vi "VNAconsole.vi"() -> ()   [LabVIEW 2017]
uses:
  ScanTarget.ctl
  ScanPara.ctl
  Action.ctl
  InstrPara.ctl
  <vilib>/Utility/xml.llb/Write to XML File(string).vi
  <vilib>/Utility/xml.llb/Read From XML File(string).vi
  <vilib>/Utility/file.llb/Write Delimited Spreadsheet (DBL).vi
  <instrlib>/Agilent ENA Series/Agilent ENA Series.lvlib
  <instrlib>/Agilent PNA Series/Agilent PNA Series.lvlib
panel:
  out "CrntScan 2":dbl[](array[numeric]) caption="Current scan"
  in  "Panel":enum32{"Meas", "Graph"}(tab)
  out "TimeLeft":dbl
  in  "ThermalizationTime":dbl=600.0 caption="Settling\nTime (sec)"
  in  "FAA_SetT":dbl caption="FAA  Set T(K)\n ADR  0=off" min=0.0 max=10.0
  in  "LoadSettings":bool caption="Load settings?"
  in  "SettingsPath":path=path "O:/68707/BF2222/LABVIEWdata/VNA" caption="Settings path"
  in  "Comment":string
  in  "Config":enum32{"PNA", "ENA"}(tab)
  in  "PNA Config":T1={"Sweep Type"=0, "Sweep Gen Type"=0, "Sweep Points"=32001, "Bandwidth (Hz)"=1000.0, "Center Freq (Hz)"=25005000000.0, "Span Freq (Hz)"=49990000000.0, "Power Level (dBm)"=-87.0, "Average Count"=1, "Electrical Delay (s)"=0.0} {"Electrical Delay (s)" min=0.0 max=1000000000.0 format="%.6p"; "Average Count" min=1 max=65536 step=1; "Power Level (dBm)" min=-87.0 max=10.0 format="%.2p"; "Span Freq (Hz)" min=0.0 max=49990000000.0 format="%.6p"; "Center Freq (Hz)" min=10000000.0 max=50000000000.0 format="%.6p"; "Bandwidth (Hz)" min=1.0 max=40000.0 format="%.2p"; "Sweep Points" min=1 max=32001 step=1; "Sweep Gen Type" items=["Analog", "Stepped"]; "Sweep Type" items=["Linear Frequency", "Log Frequency", "Power Sweep", "CW Time"]}
  in  "ENAConfig":T2={"Sweep Type"=0, "Sweep Mode"=1, "Sweep Points"=3201, "Average count"=1, "IF Bandwidth (Hz)"=1000.0, "Power Level (dBm)"=-85.0, "Center Freq (Hz)"=10000150000.0, "Span Freq (Hz)"=19999700000.0, "Electrical Delay (s)"=0.0} caption="ENA Config" {"Electrical Delay (s)" min=0.0 max=10.0 format="%.2p"; "Span Freq (Hz)" min=0.0 max=19999700000.0 format="%.6p"; "Center Freq (Hz)" min=300000.0 max=20000000000.0 format="%.6p"; "Power Level (dBm)" min=-85.0 max=10.0 format="%^.2g"; "IF Bandwidth (Hz)" min=10.0 max=1500000.0 format="%.1p"; "Average count" min=1 max=999 step=1; "Sweep Points" min=1 max=3201 step=1; "Sweep Mode" items=["Stepped", "Swept", "Fast Stepped Mode", "Fast Swept Mode"]; "Sweep Type" items=["Linear Sweep", "Logarithmic Sweep", "Segment Sweep", "Power Sweep", "DC Bias"]}
  in  "Run":bool caption="Run?"
  in  "Scans":T5(array[cluster])=[{"Target"=enum."VNA", "Parameter"=enum."N.A.", "Start"=0.0, "Stop"=0.0, "#Steps"=1, "ScanArray"=[0.0]}] {"Stop" format="%.9f"; "Start" format="%.9f"; "#Steps" min=1 step=1}
  in  "SYS":T6={"ScanStep"=[], "ScanSizes"=[], "Data Path"=path "C:/data", "Scans"=[], "GPIB_ENA"="GPIB0::17::INSTR", "Savingfolder"=path "", "GPIB_PNA"="GPIB0::16::INSTR", "PhysCH"={"Fridge"="ADR", "VNA"="PNA #E8364C"}, "GPIB_PPMS"="GPIB0::15::INSTR"} {"Scans"."Stop" format="%.9f"; "Scans"."Start" format="%.9f"}
  out "VNA Data":dbl[][](array[numeric])
  out "VNA Freq":dbl[](array[numeric])
  out "Routing":variant=variant(enum16{"Startup", "Shutdown", "SaveSettings", "LoadSettings", "InitVNA", "CloseVNA", "InitScan", "IncrementScan", "StopScan", "Target=VNA", "Acquire", "Graph", "PNA", "ENA"} enum."Graph")
  in  "Acquiring":bool
  out "Shutdown":bool=TRUE
  in  "Meas":T7={"S11"=FALSE, "S12"=FALSE, "S21"=TRUE, "S22"=FALSE}
  out "T_status":string caption="Temperature Status"
  out "FinalT":dbl
  out "ENA Mag":cluster{dbl[], "Data":dbl[]}[](graph) caption="ENA Magnitude"
  out "ENA Phz":cluster{dbl[], "Data":dbl[]}[](graph) caption="ENA Phase"
  out "CrntScan":dbl[](array[numeric]) caption="Current scan"
  out "XY Graph":cluster{"all rows":dbl[], dbl[]}[](graph)
  out "rotated and translated circle":cluster{dbl[], dbl[]}(graph)
  out "Fits":T8 {"Q_i" format="%#.0f"; "Q_c" format="%#.0f"; "Q_r" format="%#1.0f"; "f_r" format="%#_9p"}
  # "Target"
  # "Parameter"
  # "Start"
  # "Stop"
  # "Yellow fields are controls.\nBlue fields are indicators.\nCheck all yellow fields before RUN.\nScans override Config."
  # "#Steps"
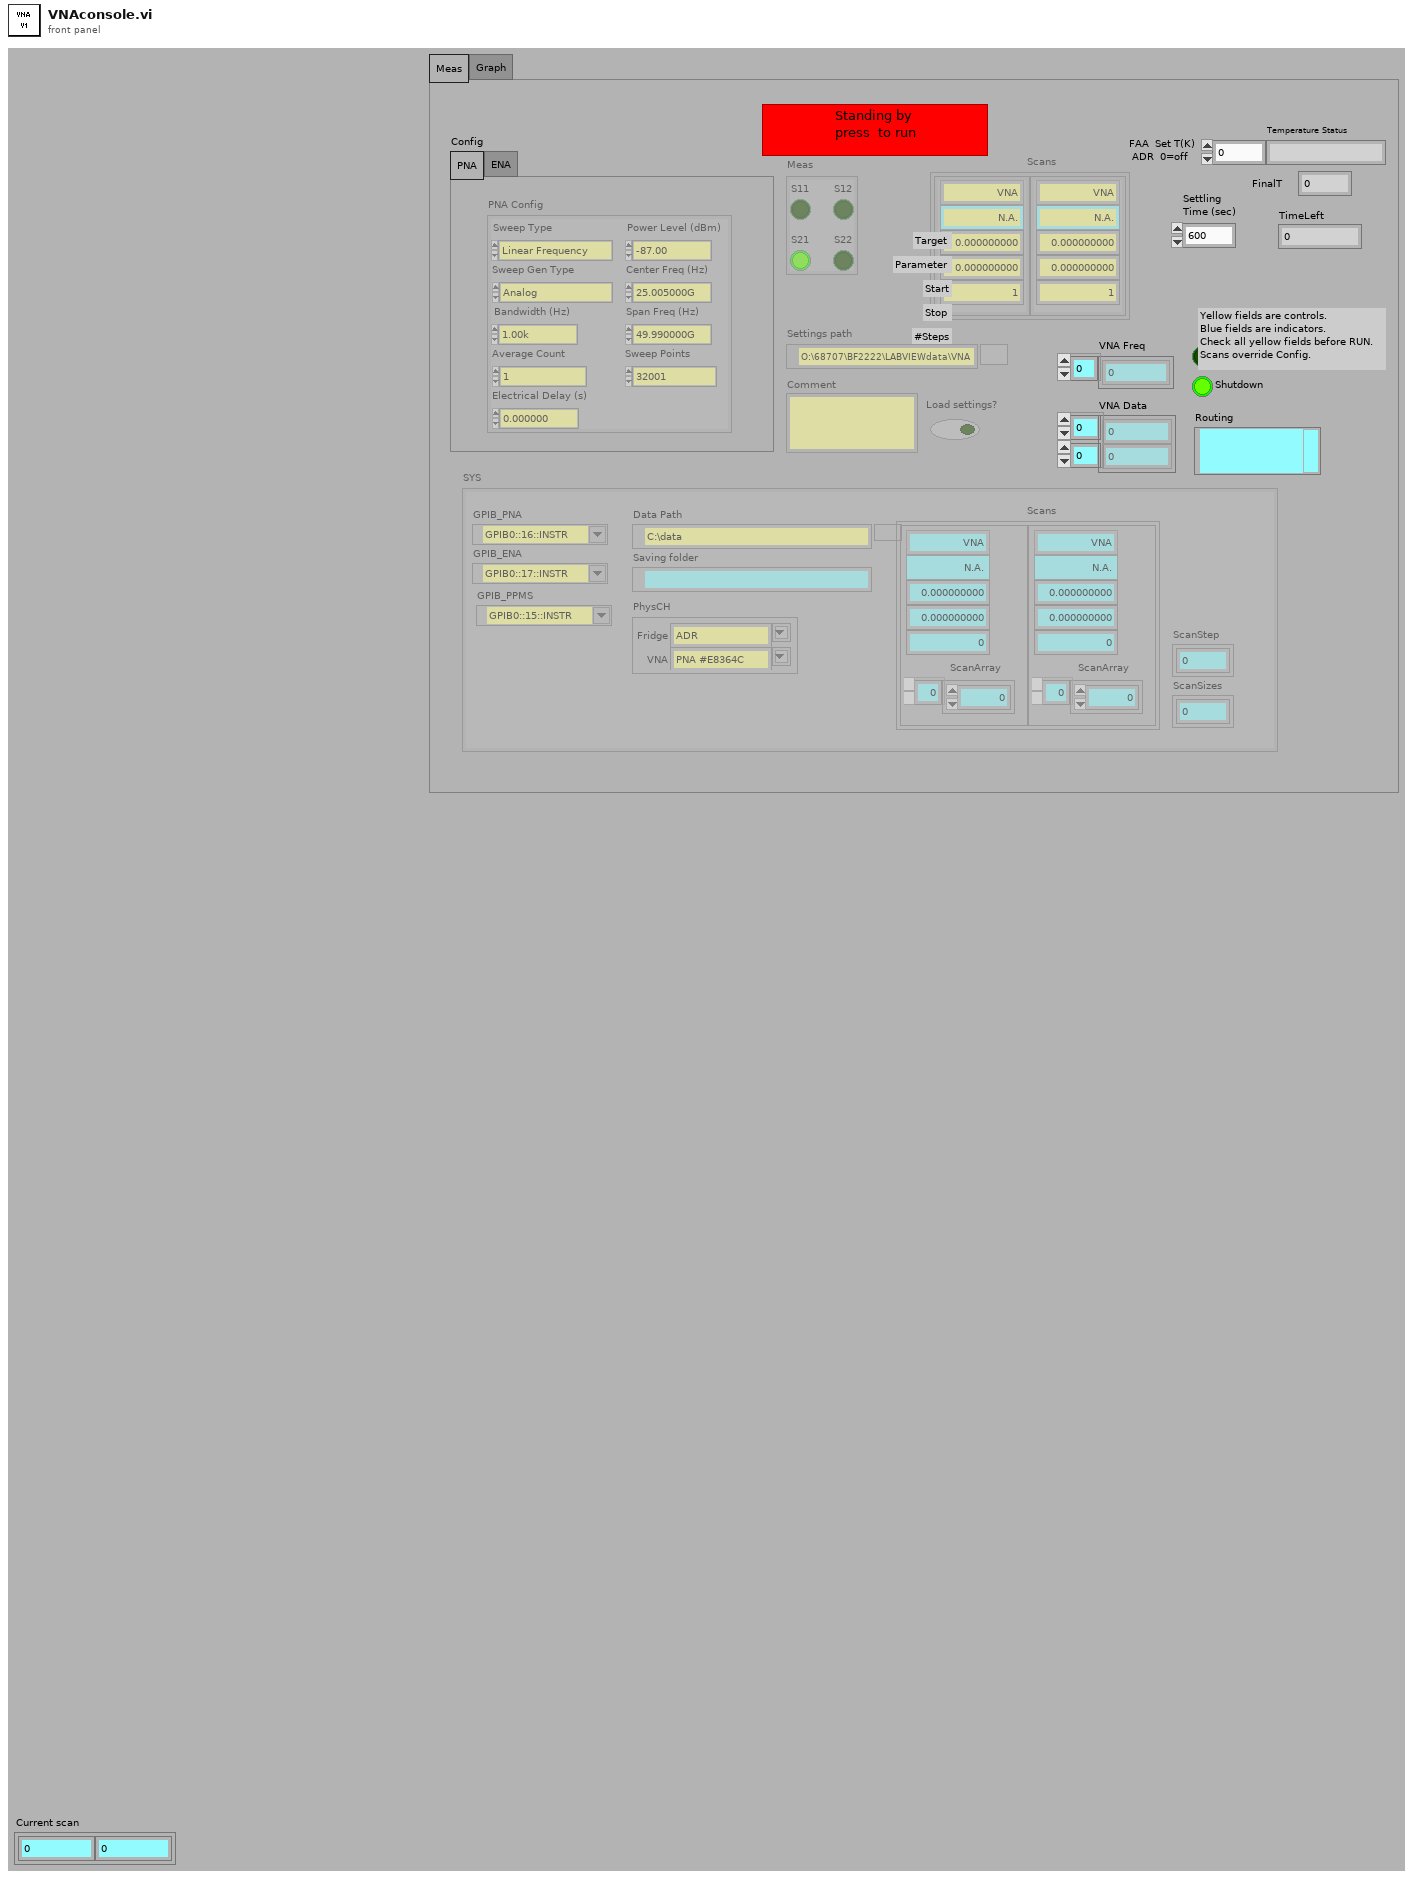
[diagram p1: front panel]
types:
  T1 = cluster{"Sweep Type":i32, "Sweep Gen Type":i32, "Sweep Points":i32, "Bandwidth (Hz)":dbl, "Center Freq (Hz)":dbl, "Span Freq (Hz)":dbl, "Power Level (dBm)":dbl, "Average Count":i32, "Electrical Delay (s)":dbl}
  T2 = cluster{"Sweep Type":u16, "Sweep Mode":u16, "Sweep Points":i32, "Average count":i32, "IF Bandwidth (Hz)":dbl, "Power Level (dBm)":dbl, "Center Freq (Hz)":dbl, "Span Freq (Hz)":dbl, "Electrical Delay (s)":dbl}
  T3 = typedef "ScanTarget.ctl" = enum16{"VNA", "Refrigerator"}
  T4 = typedef "ScanPara.ctl" = enum16{"Freq (GHz)", "Pwr (dBm)", "Temp (K)", "N.A."}
  T5 = cluster{"Target":T3, "Parameter":T4, "Start":dbl, "Stop":dbl, "#Steps":u32, "ScanArray":dbl[]}[]
  T6 = cluster{"ScanStep":i32[], "ScanSizes":i32[], "Data Path":path, "Scans":cluster{"Target":T3, "Parameter":T4, "Start":dbl, "Stop":dbl, "#Steps":u32, "ScanArray":dbl[]}[], "GPIB_ENA":refnum<visa-resource-name>, "Savingfolder":path, "GPIB_PNA":refnum<visa-resource-name>, "PhysCH":cluster{"Fridge":string, "VNA":string}, "GPIB_PPMS":refnum<visa-resource-name>}
  T7 = cluster{"S11":bool, "S12":bool, "S21":bool, "S22":bool}
  T8 = cluster{"f_r":dbl, "Q_r":dbl, "Q_c":dbl, "Q_i":dbl, "angle":dbl, "residue":dbl}
  T9 = typedef "Action.ctl" = enum16{"Startup", "Shutdown", "SaveSettings", "LoadSettings", "InitVNA", "CloseVNA", "InitScan", "IncrementScan", "StopScan", "Target=VNA", "Target=Refrigerator", "Acquire", "Graph", "PNA", "ENA", "ADR", "PPMS"}
  T10 = typedef "Semaphore RefNum" = refnum<k1>
  T11 = typedef "InstrPara.ctl" = cluster{"Parameter":string, "Channel":i32, "Instr#":i32, "Settings":variant}
  T12 = cluster{"PNA Config":cluster{"Sweep Type":i32, "Sweep Gen Type":i32, "Sweep Points":i32, "Bandwidth (Hz)":dbl, "Center Freq (Hz)":dbl, "Span Freq (Hz)":dbl, "Power Level (dBm)":dbl, "Average Count":i32, "Electrical Delay (s)":dbl}, "Meas":cluster{"S11":bool, "S12":bool, "S21":bool, "S22":bool}}
  T13 = cluster{"ENAConfig":cluster{"Sweep Type":u16, "Sweep Mode":u16, "Sweep Points":i32, "Average count":i32, "IF Bandwidth (Hz)":dbl, "Power Level (dBm)":dbl, "Center Freq (Hz)":dbl, "Span Freq (Hz)":dbl, "Electrical Delay (s)":dbl}, "Meas":cluster{"S11":bool, "S12":bool, "S21":bool, "S22":bool}}
  T14 = enum8{"Enabled", "Disabled", "Disabled and Grayed Out"}
  T15 = cluster{"Scans":cluster{"Scans":cluster{"Target":T3, "Parameter":T4, "Start":dbl, "Stop":dbl, "#Steps":u32, "ScanArray":dbl[]}[], "ScanSizes":i32[]}, "VNA":cluster{"PNA Config":cluster{"Sweep Type":i32, "Sweep Gen Type":i32, "Sweep Points":i32, "Bandwidth (Hz)":dbl, "Center Freq (Hz)":dbl, "Span Freq (Hz)":dbl, "Power Level (dBm)":dbl, "Average Count":i32, "Electrical Delay (s)":dbl}, "ENAConfig":cluster{"Sweep Type":u16, "Sweep Mode":u16, "Sweep Points":i32, "Average count":i32, "IF Bandwidth (Hz)":dbl, "Power Level (dBm)":dbl, "Center Freq (Hz)":dbl, "Span Freq (Hz)":dbl, "Electrical Delay (s)":dbl}, "Meas":cluster{"S11":bool, "S12":bool, "S21":bool, "S22":bool}}, "PhysCH":cluster{"Fridge":string, "VNA":string}, "Comment":string}
  T16 = cluster{"PNA Config":cluster{"Sweep Type":i32, "Sweep Gen Type":i32, "Sweep Points":i32, "Bandwidth (Hz)":dbl, "Center Freq (Hz)":dbl, "Span Freq (Hz)":dbl, "Power Level (dBm)":dbl, "Average Count":i32, "Electrical Delay (s)":dbl}, "ENAConfig":cluster{"Sweep Type":u16, "Sweep Mode":u16, "Sweep Points":i32, "Average count":i32, "IF Bandwidth (Hz)":dbl, "Power Level (dBm)":dbl, "Center Freq (Hz)":dbl, "Span Freq (Hz)":dbl, "Electrical Delay (s)":dbl}, "Meas":cluster{"S11":bool, "S12":bool, "S21":bool, "S22":bool}}
  T17 = cluster{"Scans":cluster{"Target":T3, "Parameter":T4, "Start":dbl, "Stop":dbl, "#Steps":u32, "ScanArray":dbl[]}[], "ScanSizes":i32[]}
  T18 = cluster{"PNA Config":variant, "Meas":cluster{"S11":bool, "S12":bool, "S21":bool, "S22":bool}}
  T19 = cluster{"Target":T3, "Parameter":T4, "Start":dbl, "Stop":dbl, "#Steps":u32, "ScanArray":dbl[]}
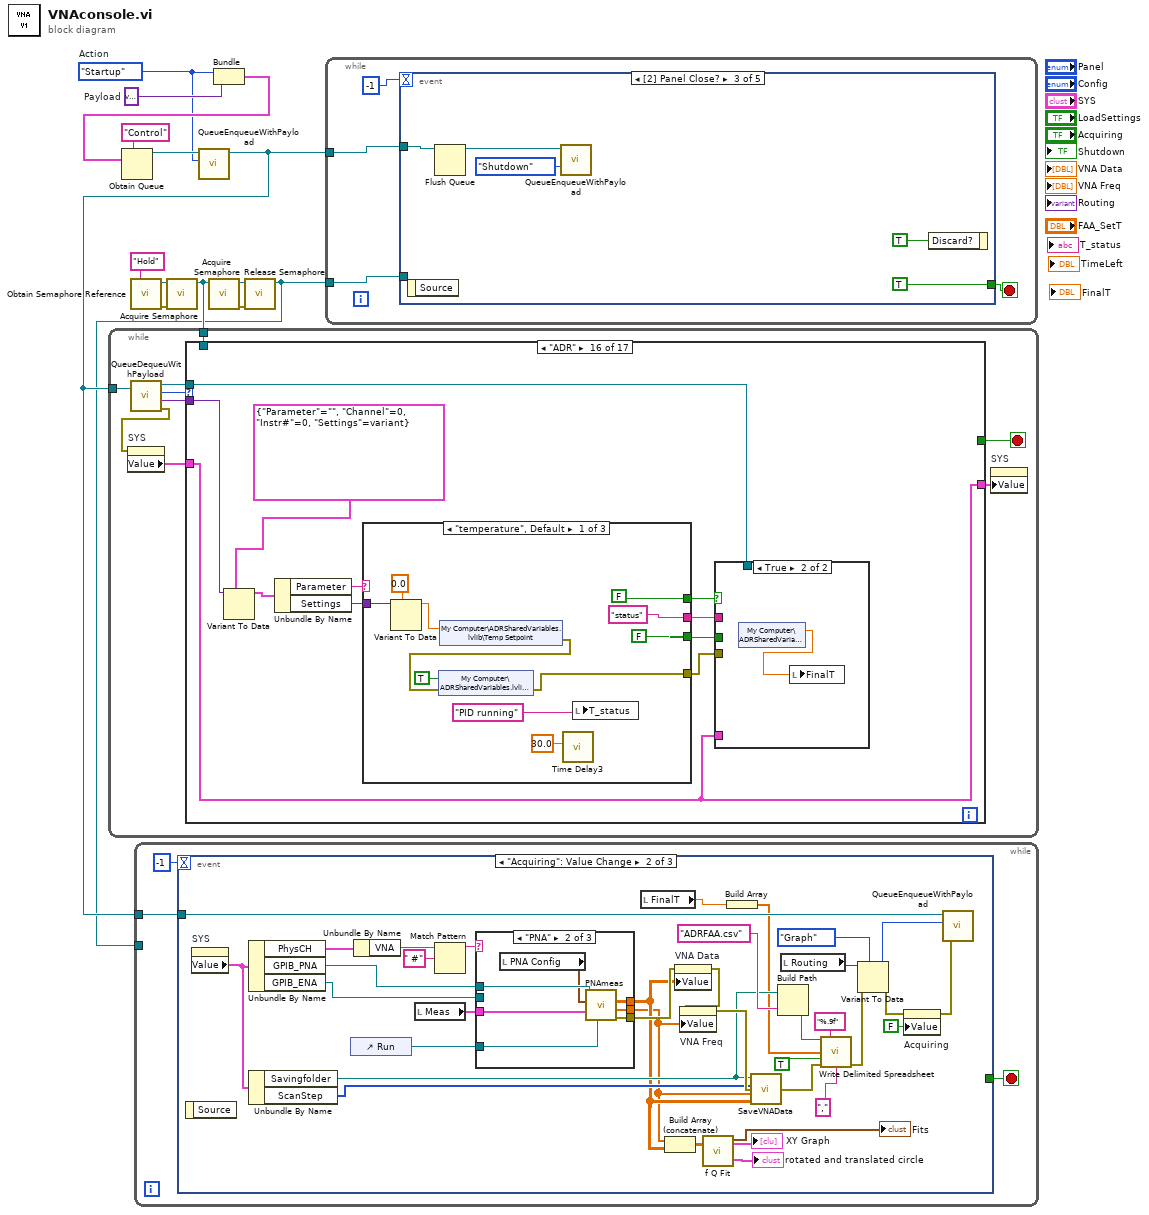
[diagram p0: block diagram]
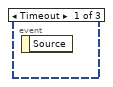
[diagram p2: hidden frame]
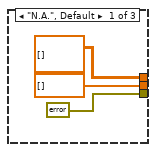
[diagram p3: hidden frame]
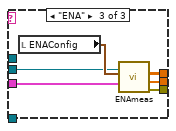
[diagram p4: hidden frame]
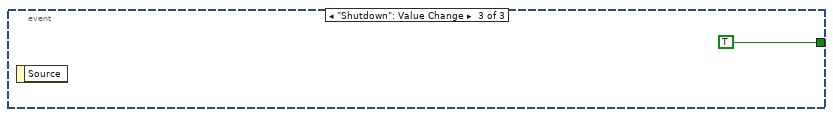
[diagram p5: hidden frame]
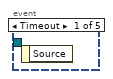
[diagram p6: hidden frame]
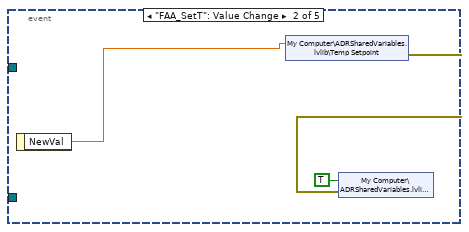
[diagram p7: hidden frame]
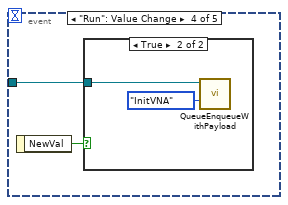
[diagram p8: hidden frame]
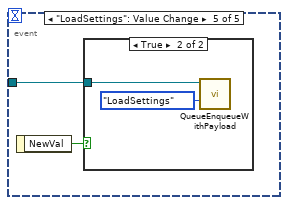
[diagram p10: hidden frame]
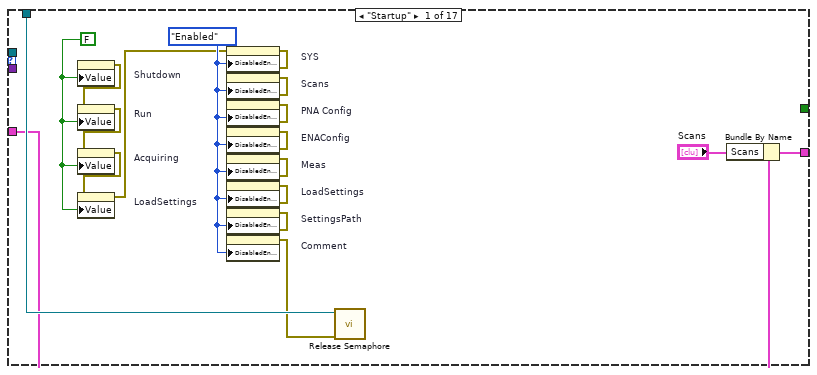
[diagram p12: hidden frame]
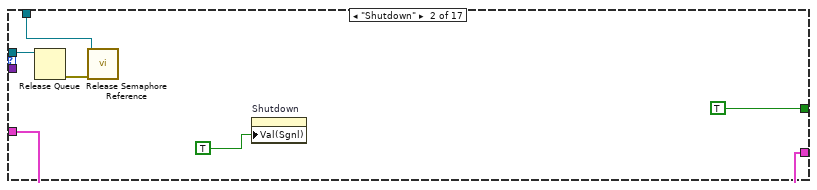
[diagram p13: hidden frame]
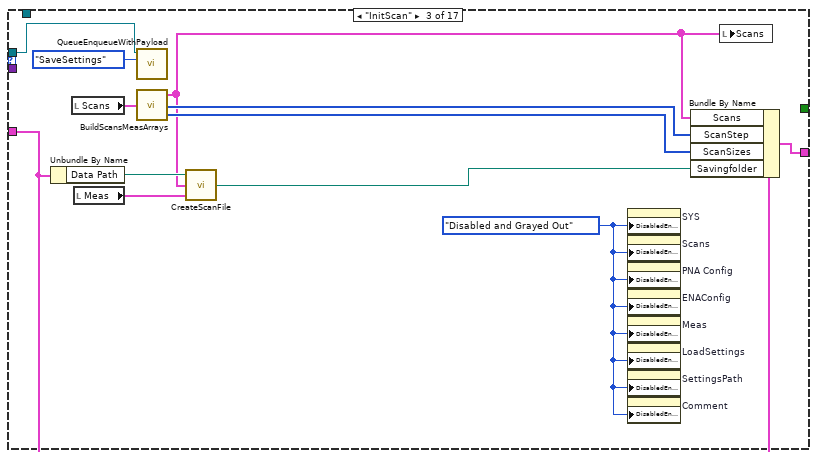
[diagram p14: hidden frame]
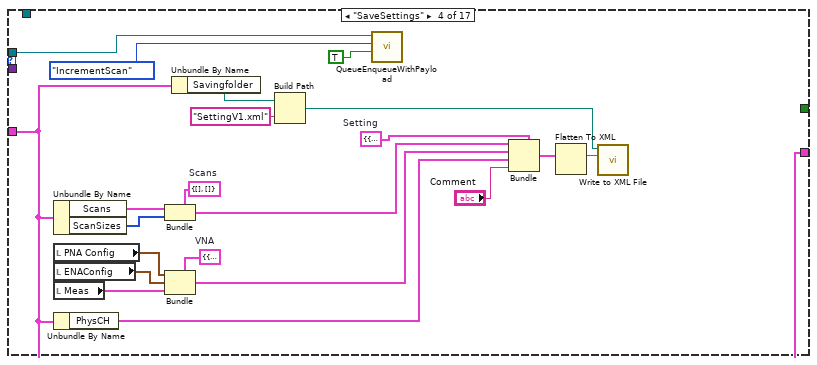
[diagram p15: hidden frame]
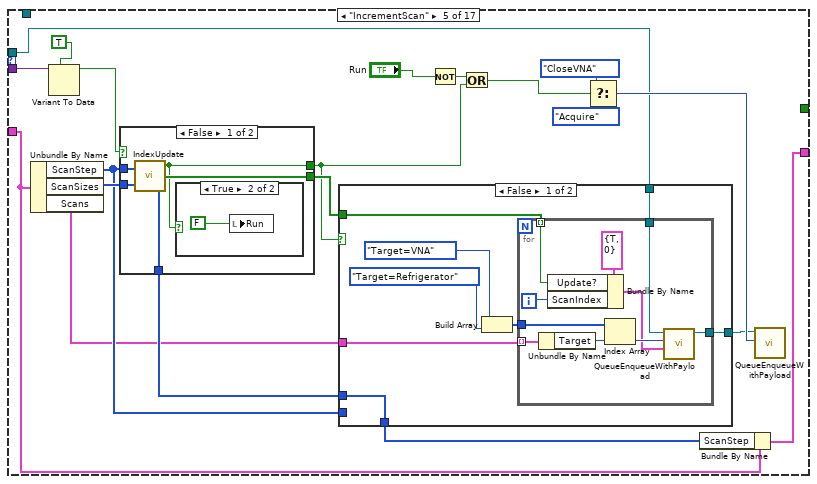
[diagram p16: hidden frame]
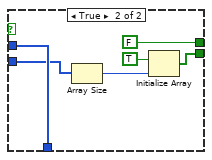
[diagram p19: hidden frame]
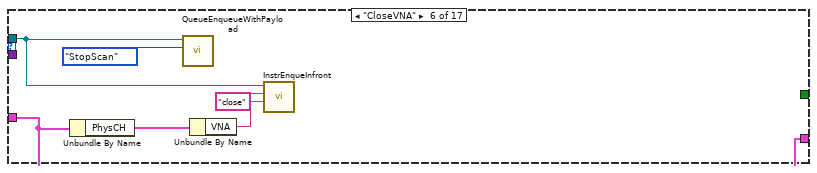
[diagram p20: hidden frame]
diagram:
  w6 = variant  # Payload
  w3 = Action."Startup"  # Action
  n1 = call <vilib>:"Obtain Semaphore Reference.vi"("name (unnamed)"="Hold") -> ("error out"=w11:errorcluster, "semaphore"=w10:T10)  [unwired: 4 in, 1 out]
  n2 = call <vilib>:"Acquire Semaphore.vi"("error in (no error)"=w11, "semaphore"=w10) -> ("semaphore out"=w9:T10)  [unwired: 3 in, 2 out]
  n3 = call <vilib>:"Acquire Semaphore.vi"("semaphore"=w9) -> ("error out"=w8:errorcluster, "semaphore out"=w7:T10)  [unwired: 4 in, 1 out]
  n4 = Bundle("Action"=w3, "Payload"=w6) -> (w5:cluster{"Action":T9, "Payload":variant})  [unwired: 1 in]
  n5 = Obtain Queue(name (unnamed)="Control", element data type=w5) -> (queue out=w4:refnum<queue>)  [unwired: 3 in, 2 out]
  n6 = call "QueueEnqueueWithPayload.vi"("Action"=w3, "Queue in"=w4) -> ("Queue out"=w2:refnum<queue>)  [unwired: 2 in, 1 out]
  n7 = while {
    tunnel: w2 -> [w16]
    tunnel: w9 -> [w21]
    stop <- w22 stop-if-true
    n8 = call "QueueDequeuWithPayload.vi"("Queue in"=w16) -> ("Queue out"=w17:refnum<queue>, "Action"=w18:T9, "Payload"=w15:variant, "error out"=w14:errorcluster)  [unwired: 1 in]
    n9 = property on="SYS" class="Clust (strict)"(error in=w14) -> ("Value"=w20:T6)  [unwired: 1 in, 2 out]
    n10 = case shown="\"ADR\"" w18 {
      tunnel: w17 -> [_ w43 w47 w76 w83 w134 _ w144 w182 w191 _ w214 w239 _ _ w309 w369]
      tunnel: [_ TRUE _ _ _ _ _ _ _ _ _ _ _ _ _ _ _] -> w22
      tunnel: w20 -> [w39 w42 w49 w72 w98 w135 w138 w147 w184 w190 w200 w209 w238 w262 w282 w311 w366]
      tunnel: [w38 w42 w50 w72 w97 w135 w138 w147 w184 w190 w199 w209 w238 w262 w282 w311 w366] -> w19
      tunnel: w21 -> [w40 w45 _ _ _ _ _ _ _ _ _ _ _ _ _ _ _]
      tunnel: w15 -> [_ _ _ _ w82 _ _ _ _ _ _ w215 w237 w263 w284 w312 w370]
      frame "Startup" {
        w34 = T14."Enabled" ("Disabled")
        w23 = FALSE ("Run")
        n11 = property on="Shutdown" class="Bool (strict)"("Value"=w23) -> (error out=w37:errorcluster)  [unwired: 2 in, 1 out]
        n12 = property on="Run" class="Bool (strict)"(error in=w37, "Value"=w23) -> (error out=w36:errorcluster)  [unwired: 1 in, 1 out]
        n13 = property on="Acquiring" class="Bool (strict)"(error in=w36, "Value"=w23) -> (error out=w25:errorcluster)  [unwired: 1 in, 1 out]
        n14 = property on="LoadSettings" class="Bool (strict)"(error in=w25, "Value"=w23) -> (error out=w24:errorcluster)  [unwired: 1 in, 1 out]
        n15 = property on="SYS" class="Clust (strict)"(error in=w24, "DisabledEnum"=w34) -> (error out=w33:errorcluster)  [unwired: 1 in, 1 out]
        n16 = property on="Scans" class="Arr (strict)"(error in=w33, "DisabledEnum"=w34) -> (error out=w32:errorcluster)  [unwired: 1 in, 1 out]
        n17 = property on="PNA Config" class="Clust (strict)"(error in=w32, "DisabledEnum"=w34) -> (error out=w31:errorcluster)  [unwired: 1 in, 1 out]
        n18 = property on="ENAConfig" class="Clust (strict)"(error in=w31, "DisabledEnum"=w34) -> (error out=w30:errorcluster)  [unwired: 1 in, 1 out]
        n19 = property on="Meas" class="Clust (strict)"(error in=w30, "DisabledEnum"=w34) -> (error out=w29:errorcluster)  [unwired: 1 in, 1 out]
        n20 = property on="LoadSettings" class="Bool (strict)"(error in=w29, "DisabledEnum"=w34) -> (error out=w28:errorcluster)  [unwired: 1 in, 1 out]
        n21 = property on="SettingsPath" class="Path"(error in=w28, "DisabledEnum"=w34) -> (error out=w27:errorcluster)  [unwired: 1 in, 1 out]
        n22 = property on="Comment" class="Str"(error in=w27, "DisabledEnum"=w34) -> (error out=w26:errorcluster)  [unwired: 1 in, 1 out]
        n23 = call <vilib>:"Release Semaphore.vi"("error in (no error)"=w26, "semaphore"=w40) -> ()  [unwired: 4 in, 2 out]
        n24 = Bundle By Name(cluster=w39, "Scans"="Scans") -> (w38:T6)
      }
      frame "Shutdown" {
        n25 = Release Queue(queue=w43) -> (error out=w44:errorcluster)  [unwired: 2 in, 2 out]
        n26 = call <vilib>:"Release Semaphore Reference.vi"("error in (no error)"=w44, "semaphore"=w45) -> ()  [unwired: 8 in, 2 out]
        n27 = property on="Shutdown" class="Bool (strict)"("Val(Sgnl)"=TRUE ("Value (Signaling)")) -> ()  [unwired: 2 in, 2 out]
      }
      frame "InitScan" {
        w48 = T14."Disabled and Grayed Out" ("Disabled")
        n28 = Unbundle By Name(w49) -> ("Data Path"=w55:path)
        n29 = local read "Scans"() -> (w56:T5)
        n30 = local read "Meas"() -> (w57:T7)
        n31 = call "QueueEnqueueWithPayload.vi"("Action"=Action."SaveSettings", "Queue in"=w47) -> ()  [unwired: 2 in, 2 out]
        n32 = call "BuildScansMeasArrays.vi"("Scans in"=w56) -> ("Scans out"=w51:T5, "ScanStep"=w58:i32[], "ScanSizes"=w53:i32[])
        n33 = call "CreateScanFile.vi"("Meas"=w57, "Scans"=w51, "PathIn"=w55) -> ("PathOut"=w54:path)
        n34 = property on="SYS" class="Clust (strict)"("DisabledEnum"=w48) -> ()  [unwired: 2 in, 2 out]
        n35 = property on="Scans" class="Arr (strict)"("DisabledEnum"=w48) -> ()  [unwired: 2 in, 2 out]
        n36 = property on="PNA Config" class="Clust (strict)"("DisabledEnum"=w48) -> ()  [unwired: 2 in, 2 out]
        n37 = property on="ENAConfig" class="Clust (strict)"("DisabledEnum"=w48) -> ()  [unwired: 2 in, 2 out]
        n38 = property on="Meas" class="Clust (strict)"("DisabledEnum"=w48) -> ()  [unwired: 2 in, 2 out]
        n39 = property on="LoadSettings" class="Bool (strict)"("DisabledEnum"=w48) -> ()  [unwired: 2 in, 2 out]
        n40 = property on="SettingsPath" class="Path"("DisabledEnum"=w48) -> ()  [unwired: 2 in, 2 out]
        n41 = property on="Comment" class="Str"("DisabledEnum"=w48) -> ()  [unwired: 2 in, 2 out]
        n42 = Bundle By Name(cluster=w49, "Scans"=w51, "ScanStep"=w58, "ScanSizes"=w53, "Savingfolder"=w54) -> (w50:T6)
        n43 = local write "Scans"(w51) -> ()
      }
      frame "SaveSettings" {
        w61 = T15 {"Scans"={"Scans"=[], "ScanSizes"=[]}, "VNA"={"PNA Config"={"Sweep Type"=0, "Sweep Gen Type"=0, "Sweep Points"=0, "Bandwidth (Hz)"=0.0, "Center Freq (Hz)"=0.0, "Span Freq (Hz)"=0.0, "Power Level (dBm)"=0.0, "Average Count"=0, "Electrical Delay (s)"=0.0}, "ENAConfig"={"Sweep Type"=0, "Sweep Mode"=0, "Sweep Points"=0, "Average count"=0, "IF Bandwidth (Hz)"=0.0, "Power Level (dBm)"=0.0, "Center Freq (Hz)"=0.0, "Span Freq (Hz)"=0.0, "Electrical Delay (s)"=0.0}, "Meas"={"S11"=FALSE, "S12"=FALSE, "S21"=FALSE, "S22"=FALSE}}, "PhysCH"={"Fridge"="", "VNA"=""}, "Comment"=""}  # Setting
        w66 = T16 {"PNA Config"={"Sweep Type"=0, "Sweep Gen Type"=0, "Sweep Points"=0, "Bandwidth (Hz)"=0.0, "Center Freq (Hz)"=0.0, "Span Freq (Hz)"=0.0, "Power Level (dBm)"=0.0, "Average Count"=0, "Electrical Delay (s)"=0.0}, "ENAConfig"={"Sweep Type"=0, "Sweep Mode"=0, "Sweep Points"=0, "Average count"=0, "IF Bandwidth (Hz)"=0.0, "Power Level (dBm)"=0.0, "Center Freq (Hz)"=0.0, "Span Freq (Hz)"=0.0, "Electrical Delay (s)"=0.0}, "Meas"={"S11"=FALSE, "S12"=FALSE, "S21"=FALSE, "S22"=FALSE}}  # VNA
        w68 = T17 {"Scans"=[], "ScanSizes"=[]}  # Scans
        n44 = Unbundle By Name(w72) -> ("Scans"=w78:T5, "ScanSizes"=w77:i32[])
        n45 = local read "PNA Config"() -> (w67:T1)
        n46 = local read "ENAConfig"() -> (w74:T2)
        n47 = local read "Meas"() -> (w73:T7)
        n48 = Unbundle By Name(w72) -> ("PhysCH"=w69:cluster{"Fridge":string, "VNA":string})
        n49 = Bundle(cluster=w68, "Scans"=w78, "ScanSizes"=w77) -> (w71:T17)
        n50 = Bundle(cluster=w66, "PNA Config"=w67, "ENAConfig"=w74, "Meas"=w73) -> (w65:T16)
        n51 = Unbundle By Name(w72) -> ("Savingfolder"=w63:path)
        n52 = Build Path(base path=w63, name or relative path="SettingV1.xml") -> (appended path=w75:path)
        n53 = call "QueueEnqueueWithPayload.vi"("Payload"=TRUE, "Action"=Action."IncrementScan", "Queue in"=w76) -> ()  [unwired: 1 in, 2 out]
        n54 = Bundle(cluster=w61, "Scans"=w71, "VNA"=w65, "PhysCH"=w69, "Comment"="Comment") -> (w60:T15)
        n55 = Flatten To XML(anything=w60) -> (xml string=w79:string)
        n56 = call-poly <vilib>:"Write to XML File.vi"("XML Input"=w79, "XML File Path"=w75) -> ()  [unwired: 7 in, 3 out]
      }
      frame "IncrementScan" {
        n57 = Unbundle By Name(w98) -> ("ScanStep"=w87:i32[], "ScanSizes"=w99:i32[], "Scans"=w86:T5)
        n58 = Variant To Data(type=TRUE, Variant=w82) -> (data=w80:bool)  [unwired: 1 in, 1 out]
        n59 = case shown="False" w80 {
          tunnel: w99 -> [w124 w128]
          tunnel: w87 -> [w120 w130]
          tunnel: [w121 FALSE ("Done")] -> w85
          tunnel: [w123 w130] -> w89
          tunnel: [w122 w126] -> w90
          frame False {
            n60 = call "IndexUpdate.vi"("ScanStepIn"=w120, "ScanSizes"=w124) -> ("Done"=w121:bool, "Update?"=w122:bool[], "ScanStepOut"=w123:i32[])
            n61 = case shown="True" w121 {
              frame False {
              }
              frame True {
                n62 = local write "Run"(FALSE ("RunScans")) -> ()
              }
            }
          }
          frame True {
            n63 = Array Size(array=w128) -> (size(s)=w129:i32)
            n64 = Initialize Array(TRUE ("Done"), w129) -> (w126:bool[])
          }
        }
        n65 = case shown="False" w85 {
          tunnel: w86 -> [w107 _]
          tunnel: w83 -> [w106 w119]
          tunnel: [w104 w119] -> w91
          tunnel: w90 -> [w103 _]
          tunnel: w89 -> [w102 _]
          tunnel: [w102 w118] -> w88
          tunnel: w87 -> [_ w118]
          frame False {
            n66 = Build Array(Action."Target=VNA" ("element"), Action."Target=Refrigerator" ("element")) -> (w105:T9[])
            n67 = for {
              tunnel: w107 -> [w114] mode=indexing
              tunnel: w105 -> [w117]
              tunnel: w106 -> [w115]
              tunnel: [w113] -> w104
              tunnel: w103 -> [w110] mode=indexing
              i -> [w109]
              n68 = Unbundle By Name(w114) -> ("Target"=w116:T3)
              n69 = Bundle By Name(cluster=cluster{"Update?":bool, "ScanIndex":i32} {"Update?"=TRUE, "ScanIndex"=0}, "Update?"=w110, "ScanIndex"=w109) -> (w108:cluster{"Update?":bool, "ScanIndex":i32})
              n70 = Index Array(array=w117, index=w116) -> (element=w112:T9)
              n71 = call "QueueEnqueueWithPayload.vi"("Payload"=w108, "Action"=w112, "Queue in"=w115) -> ("Queue out"=w113:refnum<queue>)  [unwired: 1 in, 1 out]
            }
          }
          frame True {
          }
        }
        n72 = Not(x="Run") -> (.not. x?=w96:bool)
        n73 = Or(x=w96, y=w85) -> (x .or. y?=w95:bool)
        n74 = Select(t=Action."CloseVNA" ("element"), s=w95, f=Action."Acquire" ("element")) -> (s? t:f=w94:T9)
        n75 = Bundle By Name(cluster=w98, "ScanStep"=w88) -> (w97:T6)
        n76 = call "QueueEnqueueWithPayload.vi"("Action"=w94, "Queue in"=w91) -> ()  [unwired: 2 in, 2 out]
      }
      frame "CloseVNA" {
        n77 = Unbundle By Name(w135) -> ("PhysCH"=w137:cluster{"Fridge":string, "VNA":string})
        n78 = call "QueueEnqueueWithPayload.vi"("Action"=Action."StopScan", "Queue in"=w134) -> ()  [unwired: 2 in, 2 out]
        n79 = Unbundle By Name(w137) -> ("VNA"=w132:string)
        n80 = call "InstrEnqueInfront.vi"("Para"="close" ("Parameter"), "PhysCH"=w132, "Queue in"=w134) -> ()  [unwired: 1 in, 1 out]
      }
      frame "Acquire" {
        n81 = property on="Routing" class="LVVar"("Value"=Action."Graph" ("element")) -> (error out=w140:errorcluster)  [unwired: 2 in, 1 out]
        n82 = call "Time Delay2"("error in (no error)"=w140, "Delay Time (s)"=0.1) -> ("error out"=w142:errorcluster)  [unwired: 9 in]
        n83 = property on="Acquiring" class="Bool (strict)"(error in=w142, "Val(Sgnl)"=TRUE ("Value (Signaling)")) -> ()  [unwired: 1 in, 2 out]
      }
      frame "Graph" {
        n84 = property on="VNA Freq" class="Arr (strict)"() -> ("Value"=w146:dbl[])  [unwired: 2 in, 2 out]
        n85 = property on="VNA Data" class="Arr (strict)"() -> ("Value"=w153:dbl[][])  [unwired: 2 in, 2 out]
        n86 = for {
          tunnel: w153 -> [w174] mode=indexing
          tunnel: [w173] -> w148 mode=indexing
          tunnel: w146 -> [w172]
          n87 = Bundle("Value"=w172, "Value"=w174) -> (w173:cluster{"Value":dbl[], "Value":dbl[]})  [unwired: 1 in]
        }
        n88 = call "QueueEnqueueWithPayload.vi"("Payload"=FALSE, "Action"=Action."IncrementScan" ("element"), "Queue in"=w144) -> ()  [unwired: 1 in, 2 out]
        n89 = for {
          shift-right: [w155] -> w151
          shift-left: cluster{"Value":dbl[], "Value":dbl[]}[] [] -> [w156]
          shift-right: [w157] -> w152
          shift-left: cluster{"Value":dbl[], "Value":dbl[]}[] [] -> [w159]
          tunnel: w148 -> [w158] mode=indexing
          i -> [w163]
          n90 = Quotient & Remainder(x=w163, y=2) -> (x-y*floor(x/y)=w161:i32)  [unwired: 1 out]
          n91 = Equal To 0?(x=w161) -> (x = 0?=w160:bool)
          n92 = case shown="False" w160 {
            tunnel: w159 -> [w167 w171]
            tunnel: w158 -> [w165 w170]
            tunnel: [w167 w169] -> w157
            tunnel: w156 -> [w166 w168]
            tunnel: [w164 w168] -> w155
            frame False {
              n93 = Build Array (concatenate)(w166, w165) -> (w164:cluster{"Value":dbl[], "Value":dbl[]}[])
            }
            frame True {
              n94 = Build Array (concatenate)(w171, w170) -> (w169:cluster{"Value":dbl[], "Value":dbl[]}[])
            }
          }
        }
        "ENA Mag" <- w152
        "ENA Phz" <- w151
      }
      frame "InitVNA" {
        n95 = Unbundle By Name(w184) -> ("PhysCH"=w183:cluster{"Fridge":string, "VNA":string})
        n96 = Unbundle By Name(w183) -> ("VNA"=w179:string)
        n97 = call "QueueEnqueueWithPayload.vi"("Action"=Action."InitScan", "Queue in"=w182) -> ()  [unwired: 2 in, 2 out]
        n98 = Match Pattern(string=w179, regular expression=" #") -> (before substring=w178:string)  [unwired: 1 in, 3 out]
        n99 = case shown="\"PNA\"" w178 {
          tunnel: [variant "PNA Config" "ENAConfig"] -> w177
          frame "N.A.", Default {
          }
          frame "PNA" {
          }
          frame "ENA" {
          }
        }
        n100 = Bundle("PNA Config"=w177, "Meas"="Meas") -> (w175:T18)  [unwired: 1 in]
        n101 = call "InstrEnqueInfront.vi"("Settings"=w175, "Para"="init" ("Parameter"), "PhysCH"=w179, "Queue in"=w182) -> ()  [unwired: 1 out]
      }
      frame "StopScan" {
        w189 = T14."Enabled" ("Disabled")
        n102 = Flush Queue(queue=w191) -> ()  [unwired: 1 in, 3 out]
        n103 = property on="SYS" class="Clust (strict)"("DisabledEnum"=w189) -> ()  [unwired: 2 in, 2 out]
        n104 = property on="Scans" class="Arr (strict)"("DisabledEnum"=w189) -> ()  [unwired: 2 in, 2 out]
        n105 = property on="PNA Config" class="Clust (strict)"("DisabledEnum"=w189) -> ()  [unwired: 2 in, 2 out]
        n106 = property on="ENAConfig" class="Clust (strict)"("DisabledEnum"=w189) -> ()  [unwired: 2 in, 2 out]
        n107 = property on="Meas" class="Clust (strict)"("DisabledEnum"=w189) -> ()  [unwired: 2 in, 2 out]
        n108 = property on="LoadSettings" class="Bool (strict)"("DisabledEnum"=w189) -> ()  [unwired: 2 in, 2 out]
        n109 = property on="SettingsPath" class="Path"("DisabledEnum"=w189) -> ()  [unwired: 2 in, 2 out]
        n110 = property on="Comment" class="Str"("DisabledEnum"=w189) -> ()  [unwired: 2 in, 2 out]
      }
      frame "LoadSettings" {
        w192 = T15 {"Scans"={"Scans"=[], "ScanSizes"=[]}, "VNA"={"PNA Config"={"Sweep Type"=0, "Sweep Gen Type"=0, "Sweep Points"=0, "Bandwidth (Hz)"=0.0, "Center Freq (Hz)"=0.0, "Span Freq (Hz)"=0.0, "Power Level (dBm)"=0.0, "Average Count"=0, "Electrical Delay (s)"=0.0}, "ENAConfig"={"Sweep Type"=0, "Sweep Mode"=0, "Sweep Points"=0, "Average count"=0, "IF Bandwidth (Hz)"=0.0, "Power Level (dBm)"=0.0, "Center Freq (Hz)"=0.0, "Span Freq (Hz)"=0.0, "Electrical Delay (s)"=0.0}, "Meas"={"S11"=FALSE, "S12"=FALSE, "S21"=FALSE, "S22"=FALSE}}, "PhysCH"={"Fridge"="", "VNA"=""}, "Comment"=""}  # Setting
        (unwired) "PNA #E8364C" ("VNA 2")
        n111 = call-poly <vilib>:"Read From XML File.vi"("XML File Path"="SettingsPath") -> ("error out"=w206:errorcluster, "XML Elements"=w207:string)  [unwired: 8 in, 1 out]
        n112 = Unflatten From XML(xml string=w207, type=w192, error in (no error)=w206) -> (value=w205:T15, error out=w202:errorcluster)
        n113 = property on="LoadSettings" class="Bool (strict)"(error in=w202, "Value"=FALSE ("LoadSettings")) -> ()  [unwired: 1 in, 2 out]
        n114 = Unbundle By Name(w205) -> ("Scans"=w204:T17, "VNA"=w201:T16, "PhysCH"=w193:cluster{"Fridge":string, "VNA":string})
        n115 = Unbundle By Name(w204) -> ("Scans"=w194:T5, "ScanSizes"=w198:i32[])
        n116 = Unbundle By Name(w201) -> ("PNA Config"=w197:T1, "ENAConfig"=w196:T2, "Meas"=w195:T7)
        n117 = local write "PNA Config"(w197) -> ()
        n118 = local write "ENAConfig"(w196) -> ()
        n119 = local write "Meas"(w195) -> ()
        n120 = local write "Scans"(w194) -> ()
        n121 = Bundle By Name(cluster=w200, "Scans"=w194, "ScanSizes"=w198, "PhysCH"=w193) -> (w199:T6)
      }
      frame "Target=VNA" {
        n122 = Variant To Data(type=cluster{"Update?":bool, "ScanIndex":i32} {"Update?"=FALSE, "ScanIndex"=0}, Variant=w215) -> (data=w212:cluster{"Update?":bool, "ScanIndex":i32})  [unwired: 1 in, 1 out]
        n123 = Unbundle By Name(w212) -> ("ScanIndex"=w210:i32, "Update?"=w211:bool)
        n124 = case shown="True" w211 {
          tunnel: w209 -> [_ w229]
          tunnel: w214 -> [_ w223]
          tunnel: w210 -> [_ w221]
          frame False {
          }
          frame True {
            n125 = Unbundle By Name(w229) -> ("PhysCH.VNA"=w218:string, "Scans"=w225:T5, "ScanStep"=w220:i32[])
            n126 = local read "CrntScan"() -> (w226:dbl[])
            n127 = Index Array(array=w225, index=w221) -> (element=w228:T19)
            n128 = Index Array(array=w220, index=w221) -> (element=w224:i32)
            n129 = Unbundle By Name(w228) -> ("Parameter"=w217:T4, "ScanArray"=w227:dbl[])
            n130 = Index Array(array=w227, index=w224) -> (element=w222:dbl)
            n131 = Replace Array Subset(array=w226, new element=w222, index=w221) -> (→"CrntScan":dbl[])
            n132 = case shown="\"Freq (GHz)\"" w217 {
              tunnel: ["" ("Para") "freq" ("Para") "pwr" ("Para")] -> w216
              frame "N.A.", Default {
              }
              frame "Freq (GHz)" {
              }
              frame "Pwr (dBm)" {
              }
            }
            n133 = call "InstrEnqueInfront.vi"("Settings"=w222, "Para"=w216, "PhysCH"=w218, "Queue in"=w223) -> ()  [unwired: 1 out]
          }
        }
      }
      frame "Target=Refrigerator" {
        n134 = Variant To Data(type=cluster{"Update?":bool, "ScanIndex":i32} {"Update?"=FALSE, "ScanIndex"=0}, Variant=w237) -> (data=w235:cluster{"Update?":bool, "ScanIndex":i32})  [unwired: 1 in, 1 out]
        n135 = Unbundle By Name(w235) -> ("ScanIndex"=w234:i32, "Update?"=w233:bool)
        n136 = case shown="True" w233 {
          tunnel: w238 -> [_ w253]
          tunnel: w239 -> [_ w244]
          tunnel: w234 -> [_ w247]
          frame False {
          }
          frame True {
            n137 = Unbundle By Name(w253) -> ("PhysCH.Fridge"=w243:string, "Scans"=w249:T5, "ScanStep"=w246:i32[])
            n138 = local read "CrntScan 2"() -> (w250:dbl[])
            n139 = Index Array(array=w249, index=w247) -> (element=w252:T19)
            n140 = Index Array(array=w246, index=w247) -> (element=w248:i32)
            n141 = Unbundle By Name(w252) -> ("Parameter"=w242:T4, "ScanArray"=w251:dbl[])
            n142 = Index Array(array=w251, index=w248) -> (element=w240:dbl)
            n143 = Replace Array Subset(array=w250, new element=w240, index=w247) -> (→"CrntScan 2":dbl[])
            n144 = case shown="\"Temp (K)\"" w242 {
              tunnel: ["" ("Para") "temperature" ("Para")] -> w241
              tunnel: w240 -> [_ w255]
              frame "N.A.", Default {
              }
              frame "Temp (K)" {
                n145 = local write "FAA_SetT"(w255) -> ()
              }
            }
            n146 = call "InstrEnqueInfront.vi"("Settings"=w240, "Para"=w241, "PhysCH"=w243, "Queue in"=w244) -> ()  [unwired: 1 out]
          }
        }
      }
      frame "PNA" {
        n147 = local read "PNA Config"() -> (w258:T1)
        n148 = Variant To Data(type=T11 {"Parameter"="", "Channel"=0, "Instr#"=0, "Settings"=variant(cluster{"Numeric":dbl} {"Numeric"=0.0})} ("output cluster"), Variant=w263) -> (data=w265:T11)  [unwired: 1 in, 1 out]
        n149 = Unbundle By Name(w262) -> ("GPIB_PNA"=w261:refnum<visa-resource-name>)
        n150 = Unbundle By Name(w265) -> ("Parameter"=w260:string, "Settings"=w259:variant)
        n151 = Unbundle By Name(w258) -> ("Span Freq (Hz)"=w257:dbl)
        n152 = case shown="\"init\"" w260 {
          tunnel: w259 -> [_ w271 w275 w280 _]
          tunnel: w261 -> [_ w267 w274 w277 w281]
          tunnel: w257 -> [_ _ w272 _ _]
          frame "N.A.", Default {
          }
          frame "init" {
            n153 = Variant To Data(type=T12 {"PNA Config"={"Sweep Type"=0, "Sweep Gen Type"=0, "Sweep Points"=0, "Bandwidth (Hz)"=0.0, "Center Freq (Hz)"=0.0, "Span Freq (Hz)"=0.0, "Power Level (dBm)"=0.0, "Average Count"=0, "Electrical Delay (s)"=0.0}, "Meas"={"S11"=FALSE, "S12"=FALSE, "S21"=FALSE, "S22"=FALSE}} ("output cluster"), Variant=w271) -> (data=w270:T12)  [unwired: 1 in, 1 out]
            n154 = Unbundle By Name(w270) -> ("PNA Config"=w268:T1, "Meas"=w266:T7)
            n155 = call "PNAinit.vi"("Meas"=w266, "PNA Config"=w268, "VISA session"=w267) -> ()  [unwired: 1 in, 2 out]
          }
          frame "freq" {
            n156 = Variant To Data(type=0.0 ("Numeric"), Variant=w275) -> (data=w273:dbl)  [unwired: 1 in, 1 out]
            n157 = call <instrlib>:"Configure Freq Center Span.vi"("Span Freq (2.9997 E+9)"=w272, "Center Freq (1.50015 E+9)"=w273, "VISA session"=w274) -> ()  [unwired: 7 in, 2 out]
          }
          frame "pwr" {
            n158 = Variant To Data(type=0.0 ("Numeric"), Variant=w280) -> (data=w278:dbl)  [unwired: 1 in, 1 out]
            n159 = call <instrlib>:"Configure Power Level.vi"("Power Level (0.0)"=w278, "VISA Resource Name"=w277) -> ()  [unwired: 8 in, 2 out]
          }
          frame "close" {
            n160 = call "PNAclose.vi"("VISA session"=w281) -> ()  [unwired: 1 in, 1 out]
          }
        }
      }
      frame "ENA" {
        n161 = Variant To Data(type=T11 {"Parameter"="", "Channel"=0, "Instr#"=0, "Settings"=variant(cluster{"Numeric":dbl} {"Numeric"=0.0})} ("output cluster"), Variant=w284) -> (data=w288:T11)  [unwired: 1 in, 1 out]
        n162 = Unbundle By Name(w288) -> ("Parameter"=w287:string, "Settings"=w285:variant)
        n163 = Unbundle By Name(w282) -> ("GPIB_ENA"=w283:refnum<visa-resource-name>)
        n164 = case shown="\"init\"" w287 {
          tunnel: w285 -> [_ w293 w298 w303 _]
          tunnel: w283 -> [_ w294 w297 w300 w304]
          frame "N.A.", Default {
          }
          frame "init" {
            n165 = Variant To Data(type=T13 {"ENAConfig"={"Sweep Type"=0, "Sweep Mode"=0, "Sweep Points"=0, "Average count"=0, "IF Bandwidth (Hz)"=0.0, "Power Level (dBm)"=0.0, "Center Freq (Hz)"=0.0, "Span Freq (Hz)"=0.0, "Electrical Delay (s)"=0.0}, "Meas"={"S11"=FALSE, "S12"=FALSE, "S21"=FALSE, "S22"=FALSE}} ("ENAsetting"), Variant=w293) -> (data=w291:T13)  [unwired: 1 in, 1 out]
            n166 = Unbundle By Name(w291) -> ("ENAConfig"=w290:T2, "Meas"=w289:T7)
            n167 = call "ENAinit.vi"("Meas"=w289, "ENA Config"=w290, "VISA session"=w294) -> ()  [unwired: 1 in, 2 out]
          }
          frame "freq" {
            w295 = u16 2 items=["Start", "Stop", "Center", "Span"] ("Stimulus (0: Start)")
            n168 = Variant To Data(type=0.0 ("Numeric"), Variant=w298) -> (data=w296:dbl)  [unwired: 1 in, 1 out]
            n169 = call <instrlib>:"Configure Sweep Stimulus.vi"("Parameter (0.0)"=w296, "Stimulus (0: Start)"=w295, "VISA resource name"=w297) -> ()  [unwired: 7 in, 2 out]
          }
          frame "pwr" {
            n170 = Variant To Data(type=0.0 ("Numeric"), Variant=w303) -> (data=w301:dbl)  [unwired: 1 in, 1 out]
            n171 = call <instrlib>:"Configure Power.vi"("VISA resource name"=w300, "Power Level (0.0)"=w301) -> ()  [unwired: 12 in, 2 out]
          }
          frame "close" {
            n172 = call "ENAclose.vi"("VISA session"=w304) -> ()  [unwired: 1 in, 1 out]
          }
        }
      }
      frame "ADR" {
        n173 = Variant To Data(type=T11 {"Parameter"="", "Channel"=0, "Instr#"=0, "Settings"=variant(cluster{"Numeric":dbl} {"Numeric"=0.0})} ("output cluster"), Variant=w312) -> (data=w315:T11)  [unwired: 1 in, 1 out]
        n174 = Unbundle By Name(w315) -> ("Parameter"=w310:string, "Settings"=w313:variant)
        n175 = case shown="\"temperature\", Default" w310 {
          tunnel: w313 -> [w331 _ w352]
          tunnel: [w327 errorcluster {"status"=FALSE, "code"=0, "source"=""} ("error IO") w348] -> w308
          tunnel: [FALSE ("Boolean") FALSE ("Boolean") w344] -> w306
          tunnel: ["status" ("Para") w338 "Thermalize" ("Para")] -> w307
          tunnel: [FALSE TRUE FALSE] -> w305
          frame "temperature", Default {
            n176 = Variant To Data(type=0.0 ("Numeric"), Variant=w331) -> (data=w330:dbl)  [unwired: 1 in, 1 out]
            n177 = shared-variable "My Computer\\ADRSharedVariables.lvlib\\Temp Setpoint"(w330) -> (error out=w329:errorcluster)  [unwired: 1 in]
            n178 = shared-variable "My Computer\\ADRSharedVariables.lvlib\\Set Temp"(TRUE ("Set Temp"), error in=w329) -> (error out=w327:errorcluster)
            n179 = call "Time Delay3"("Delay Time (s)"=30.0) -> ()  [unwired: 10 in, 1 out]
            n180 = local write "T_status"("PID running" ("T_status")) -> ()
          }
          frame "status" {
            n181 = shared-variable "My Computer\\ADRSharedVariables.lvlib\\TempStatus"() -> (w335:bool)  [unwired: 1 in, 1 out]
            n182 = local write "T_status"("PID running" ("T_status")) -> ()
            n183 = Select(t="Thermalize", s=w335, f="status" ("Para")) -> (s? t:f=w338:string)
          }
          frame "Thermalize" {
            n184 = Variant To Data(type=TRUE, Variant=w352) -> (data=w351:bool)  [unwired: 1 in, 1 out]
            n185 = call "Elapsed Time"("Time Target (s)"="ThermalizationTime", "Reset"=w351) -> ("Elapsed Time (s)"=w347:dbl, "Time has Elapsed"=w344:bool, "error out"=w348:errorcluster)  [unwired: 10 in, 5 out]
            n186 = Subtract(x="ThermalizationTime", y=w347) -> (x-y=w345:dbl)
            n187 = local write "TimeLeft"(w345) -> ()
            n188 = Select(t="Done", s=w344, f="Thermalizing" ("T_status")) -> (s? t:f=w341:string)
            n189 = local write "T_status"(w341) -> ()
          }
        }
        n190 = case shown="True" w306 {
          tunnel: w308 -> [_ _]
          tunnel: w311 -> [w319 _]
          tunnel: w309 -> [w318 _]
          tunnel: w307 -> [w316 _]
          tunnel: w305 -> [w317 _]
          frame False {
            n191 = Unbundle By Name(w319) -> ("PhysCH.Fridge"=w320:string)
            n192 = call "InstrEnqueInfront.vi"("Settings"=w317, "Para"=w316, "PhysCH"=w320, "Queue in"=w318) -> ()  [unwired: 1 out]
          }
          frame True {
            n193 = shared-variable "My Computer\\ADRSharedVariables.lvlib\\FAA"() -> (w321:dbl)  [unwired: 1 in, 1 out]
            n194 = local write "FinalT"(w321) -> ()
          }
        }
      }
      frame "PPMS" {
        n195 = Unbundle By Name(w366) -> ("Scans"=w355:T5, "GPIB_PPMS"=w359:refnum<visa-resource-name>)
        n196 = Type Cast(type="", x=w359) -> (*(type *) &x=w361:string)
        n197 = Variant To Data(type=T11 {"Parameter"="", "Channel"=0, "Instr#"=0, "Settings"=variant(cluster{"Numeric":dbl} {"Numeric"=0.0})} ("output cluster"), Variant=w370) -> (data=w373:T11)  [unwired: 1 in, 1 out]
        n198 = Index Array(array=w355) -> (element=w356:T19)  [unwired: 1 in]
        n199 = Unbundle By Name(w356) -> ("Parameter"=w357:T4)
        n200 = Unbundle By Name(w373) -> ("Parameter"=w365:string, "Settings"=w371:variant)
        n201 = Match Pattern(string=w361, regular expression="::") -> (after substring=w363:string)  [unwired: 1 in, 3 out]
        n202 = String Subset(string=w363, length (rest)=2 ("length (rest)")) -> (substring=w358:string)  [unwired: 1 in]
        n203 = case shown="\"Temp (K)\"" w357 {
          tunnel: ["" ("Para") "temperature" ("Para")] -> w354
          frame "N.A.", Default {
          }
          frame "Temp (K)" {
          }
        }
        n204 = case shown="\"status\"" w365 {
          tunnel: w371 -> [_ _ w400]
          tunnel: [errorcluster {"status"=FALSE, "code"=0, "source"=""} ("error IO") w385 w394] -> w368
          tunnel: [_ w386 FALSE] -> w367
          tunnel: w358 -> [_ w387 w399]
          tunnel: w354 -> [_ w384 _]
          frame "N.A.", Default {
            (unwired) FALSE
            (unwired) "N.A." ("Para")
            (unwired) errorcluster {"status"=FALSE, "code"=0, "source"=""} ("error out")
          }
          frame "status" {
            n205 = case shown="\"temperature\"" w384 {
              tunnel: w387 -> [_ w393]
              tunnel: [TRUE ("Temperature Stable?") w392] -> w386
              tunnel: [errorcluster {"status"=FALSE, "code"=0, "source"=""} ("error out") w391] -> w385
              frame "False", Default {
              }
              frame "temperature" {
                n206 = call <instrlib>:"PPMS temp status.vi"("GPIB address"=w393) -> ("Temperature Stable?"=w392:bool, "Temperature Status"=w390:string, "error out"=w391:errorcluster)  [unwired: 2 in, 1 out]
                n207 = local write "T_status"(w390) -> ()
              }
            }
          }
          frame "temperature" {
            n208 = Variant To Data(type=0.0 ("Numeric"), Variant=w400) -> (data=w398:dbl)  [unwired: 1 in, 1 out]
            n209 = call <instrlib>:"PPMS set temp.vi"("PPMS GPIB address"=w399, "Set Temperature"=w398, "Approach Method"=enum16{"Fast Settle", "No overshoot"}."No overshoot", "Approach Rate( 0-20)"=20.0) -> ("error out"=w395:errorcluster)  [unwired: 1 in]
            n210 = call "Time Delay"("error in (no error)"=w395) -> ("error out"=w394:errorcluster)  [unwired: 10 in]
          }
        }
        n211 = case shown="False" w367 {
          tunnel: w368 -> [w380 _]
          tunnel: w369 -> [w379 _]
          tunnel: w366 -> [w377 _]
          tunnel: w358 -> [_ w382]
          frame False {
            n212 = Unbundle By Name(w377) -> ("PhysCH.Fridge"=w378:string)
            n213 = call "InstrEnqueInfront.vi"("Settings"=w380, "Para"="status", "PhysCH"=w378, "Queue in"=w379) -> ()  [unwired: 1 out]
          }
          frame True {
            n214 = call <instrlib>:"PPMS temperature.vi"("GPIB address"=w382) -> ("Temperature (K)"=w381:dbl)  [unwired: 2 in, 1 out]
            n215 = local write "FinalT"(w381) -> ()
          }
        }
      }
    }
    n216 = property on="SYS" class="Clust (strict)"("Value"=w19) -> ()  [unwired: 2 in, 2 out]
  }
  n217 = call <vilib>:"Release Semaphore.vi"("error in (no error)"=w8, "semaphore"=w7) -> ("semaphore out"=w1:T10)  [unwired: 4 in, 1 out]
  n218 = while {
    tunnel: w2 -> [w403]
    tunnel: w1 -> [_]
    stop <- w404 stop-if-true
    n219 = event shown="[1] \"Acquiring\": Value Change" {
      selector: _ -> [_ _ _]
      dyn-events: _ -> [_ _ _]
      timeout: -1 -> [_ _ _]
      tunnel: [_ _ TRUE] -> w404
      tunnel: w403 -> [_ w440 _]
      event Timeout {
        n220 = event-data() -> ()  [unwired: 1 in, 1 out]
      }
      event "Acquiring": Value Change {
        n221 = event-data() -> ()  [unwired: 1 in, 1 out]
        n222 = property on="SYS" class="Clust (strict)"() -> ("Value"=w424:T6)  [unwired: 2 in, 2 out]
        n223 = Unbundle By Name(w424) -> ("PhysCH"=w429:cluster{"Fridge":string, "VNA":string}, "GPIB_PNA"=w436:refnum<visa-resource-name>, "GPIB_ENA"=w426:refnum<visa-resource-name>)
        n224 = Unbundle By Name(w424) -> ("Savingfolder"=w415:path, "ScanStep"=w423:i32[])
        n225 = control-ref of="Run"() -> (w413:refnum<vi>)
        n226 = Unbundle By Name(w429) -> ("VNA"=w433:string)
        n227 = local read "Meas"() -> (w432:T7)
        n228 = Match Pattern(string=w433, regular expression=" #") -> (before substring=w435:string)  [unwired: 1 in, 3 out]
        n229 = case shown="\"PNA\"" w435 {
          tunnel: w436 -> [_ w448 _]
          tunnel: w432 -> [_ w446 w456]
          tunnel: [dbl[][] [] ("ENA Data") w451 w455] -> w408
          tunnel: [dbl[] [] ("ENA Freq") w450 w454] -> w407
          tunnel: [errorcluster {"status"=FALSE, "code"=0, "source"=""} ("Error Out") w449 w453] -> w431
          tunnel: w426 -> [_ _ w452]
          tunnel: w413 -> [_ w445 _]
          frame "N.A.", Default {
          }
          frame "PNA" {
            n230 = local read "PNA Config"() -> (w447:T1)
            n231 = call "PNAmeas.vi"("Run"=w445, "Meas"=w446, "PNA Config"=w447, "VISA session"=w448) -> ("Error Out"=w449:errorcluster, "PNAfreq"=w450:dbl[], "PNAdata"=w451:dbl[][])  [unwired: 1 in, 1 out]
          }
          frame "ENA" {
            n232 = local read "ENAConfig"() -> (w457:T2)
            n233 = call "ENAmeas.vi"("Meas"=w456, "ENA Config"=w457, "VISA session"=w452) -> ("Error Out"=w453:errorcluster, "ENAfreq"=w454:dbl[], "ENAdata"=w455:dbl[][])  [unwired: 1 in, 1 out]
          }
        }
        n234 = local read "FinalT"() -> (w406:dbl)
        n235 = Build Array (concatenate)(w407, w408) -> (w409:dbl[][])
        n236 = property on="VNA Data" class="Arr (strict)"(error in=w431, "Value"=w408) -> (error out=w430:errorcluster)  [unwired: 1 in, 1 out]
        n237 = property on="VNA Freq" class="Arr (strict)"(error in=w430, "Value"=w407) -> (error out=w425:errorcluster)  [unwired: 1 in, 1 out]
        n238 = call "f Q Fit.vi"("f,Mag,Th"=w409) -> ("XY Graph"=→"XY Graph":cluster{"all rows":dbl[], dbl[]}[], "rotated and translated circle"=→"rotated and translated circle":cluster{dbl[], dbl[]}, "Fits"=→"Fits":T8)  [unwired: 3 out]
        n239 = Build Array(w406) -> (w414:dbl[])
        n240 = call "SaveVNAData.vi"("Savingfolder"=w415, "ScanStep"=w423, "VNA Freq"=w407, "VNA Data"=w408, "error in (no error)"=w425) -> ("error out"=w419:errorcluster)
        n241 = Build Path(base path=w415, name or relative path="ADRFAA.csv") -> (appended path=w417:path)
        n242 = local read "Routing"() -> (w438:variant)
        n243 = call-poly <vilib>:"Write Delimited Spreadsheet.vi"("file path (dialog if empty)"=w417, "format (%.3f)"="%.9f", "1D data"=w414, "append to file? (new file:F)"=TRUE, "error in (no error)"=w419, "delimiter (\\t)"="," ("delimiter (\\t)")) -> ("error out"=w420:errorcluster)  [unwired: 8 in, 1 out]
        n244 = Variant To Data(error in=w420, type=Action."Graph" ("element"), Variant=w438) -> (data=w427:T9, error out=w437:errorcluster)
        n245 = property on="Acquiring" class="Bool (strict)"(error in=w437, "Value"=FALSE ("Acquire")) -> (error out=w439:errorcluster)  [unwired: 1 in, 1 out]
        n246 = call "QueueEnqueueWithPayload.vi"("error in (no error)"=w439, "Action"=w427, "Queue in"=w440) -> ()  [unwired: 1 in, 2 out]
      }
      event "Shutdown": Value Change {
        n247 = event-data() -> ()  [unwired: 1 in, 1 out]
      }
    }
  }
  n248 = while {
    tunnel: w2 -> [w462]
    tunnel: w1 -> [w459]
    stop <- w460 stop-if-true
    n249 = event shown="[2] Panel Close?" {
      selector: _ -> [_ _ _ _ _]
      dyn-events: _ -> [_ _ _ _ _]
      timeout: -1 -> [_ _ _ _ _]
      tunnel: w462 -> [_ _ w468 w472 w476]
      tunnel: [_ _ TRUE _ _] -> w460
      tunnel: w459 -> [_ _ _ _ _]
      event Timeout {
        n250 = event-data() -> ()  [unwired: 2 out]
      }
      event "FAA_SetT": Value Change {
        n251 = event-data() -> ("NewVal"=w463:dbl)  [unwired: 1 out]
        n252 = shared-variable "My Computer\\ADRSharedVariables.lvlib\\Temp Setpoint"(w463) -> (error out=w465:errorcluster)  [unwired: 1 in]
        n253 = shared-variable "My Computer\\ADRSharedVariables.lvlib\\Set Temp"(TRUE ("Set Temp"), error in=w465) -> ()  [unwired: 1 out]
      }
      event Panel Close? {
        n254 = event-data() -> ()  [unwired: 2 out]
        n255 = Flush Queue(queue=w468) -> (queue out=w469:refnum<queue>)  [unwired: 1 in, 2 out]
        n256 = call "QueueEnqueueWithPayload.vi"("Action"=Action."Shutdown" ("States"), "Queue in"=w469) -> ()  [unwired: 2 in, 2 out]
        n257 = event-data("Discard?"=TRUE) -> ()  [unwired: 1 in, 1 out]
      }
      event "Run": Value Change {
        n258 = event-data() -> ("NewVal"=w471:bool)  [unwired: 1 out]
        n259 = case shown="True" w471 {
          tunnel: w472 -> [_ w473]
          frame False {
          }
          frame True {
            n260 = call "QueueEnqueueWithPayload.vi"("Action"=Action."InitVNA", "Queue in"=w473) -> ()  [unwired: 2 in, 2 out]
          }
        }
      }
      event "LoadSettings": Value Change {
        n261 = event-data() -> ("NewVal"=w475:bool)  [unwired: 1 out]
        n262 = case shown="True" w475 {
          tunnel: w476 -> [_ w477]
          frame False {
          }
          frame True {
            n263 = call "QueueEnqueueWithPayload.vi"("Action"=Action."LoadSettings", "Queue in"=w477) -> ()  [unwired: 2 in, 2 out]
          }
        }
      }
    }
  }
